vi "LCD.vi"(1 "stop":bool, 9 "Row 2":string, 10 "Row 1":string) -> ()   [LabVIEW 2017]
panel:
  out "error out":errorcluster
  in  "Back Light":bool
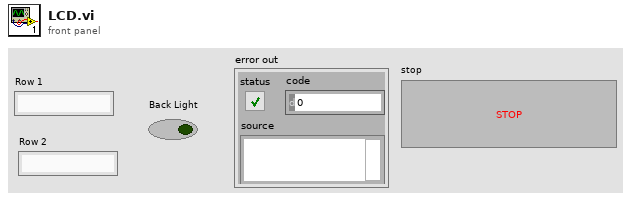
[diagram p1: front panel]
types:
  T1 = typedef "I2C.lvlib/I2C Reference.ctl" = cluster{"myRIO Reference":T2, "I2C Channels Enum":T6, "I2C Configuration":T7}
  T2 = typedef "myRIO Generic Hardware Reference.ctl" = cluster{"myRIO Model":T3, "myRIO Hardware Reference":T4}
  T3 = typedef "Hardware Version Enum.ctl" = enum16{"Unknown", "myRIO-1900", "myRIO-1950", "roboRIO", "NI ELVIS RIO CM"}
  T4 = typedef "myRIO v1.0 Reference.ctl" = cluster{"Generic FPGA Reference":T5, "Allow multiple opens":bool}
  T5 = typedef "Generic FPGA Reference.ctl" = refnum<k20>
  T6 = typedef "I2C Channels Enum.ctl" = enum16{"Not Connected", "A/I2C", "B/I2C", "I2C/I2C"}
  T7 = typedef "I2C.lvlib/I2C Configuration.ctl" = cluster{"I2C Transfer Rate":T8}
  T8 = typedef "I2C.lvlib/I2C Transfer Rate.ctl" = enum16{"Standard mode (100 kbps)", "Fast mode (400 kbps)"}
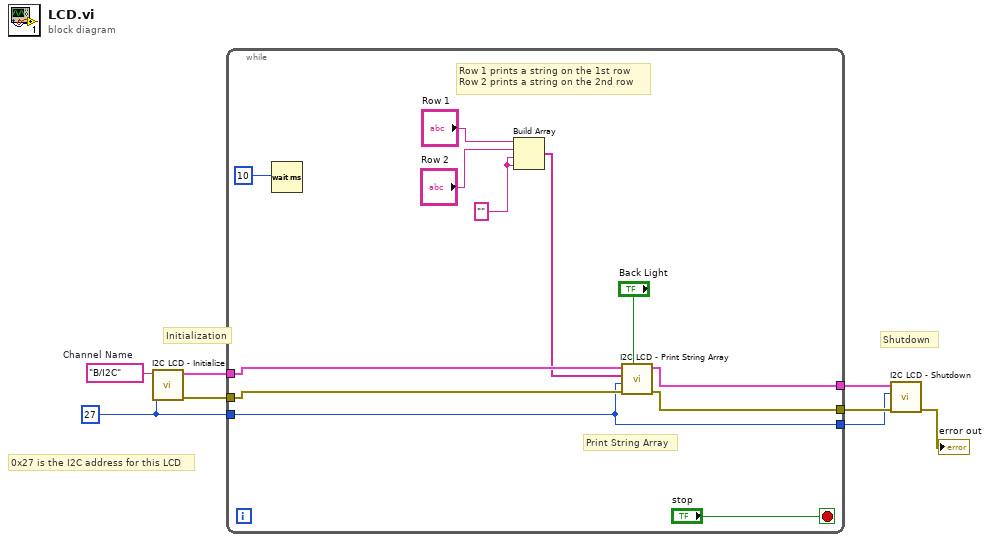
[diagram p0: block diagram]
diagram:
  w1 = tag "B/I2C"  # Channel Name
  w8 = u8 27 ("Slave Address (7-bit)")
  # "Initialization"
  # "Shutdown"
  # "0x27 is the I2C address for this LCD"
  n1 = call "I2C LCD - Initialize.vi"("Slave Address (7-bit)"=w8, "Channel Name"=w1) -> ("error out"=w7:errorcluster, "I2C Ref Out"=w6:T1)  [unwired: 8 in]
  n2 = while {
    tunnel: w8 -> [w16]
    tunnel: w7 -> [w20]
    tunnel: w6 -> [w18]
    tunnel: [w19] -> w5
    tunnel: [w17] -> w4
    tunnel: [w16] -> w3
    stop <- "stop" stop-if-true
    w11 = ""
    # "Row 1 prints a string on the 1st row\nRow 2 prints a string on the 2nd row"
    # "Print String Array"
    n3 = Wait (ms)(milliseconds to wait=10) -> ()  [unwired: 1 out]
    n4 = Build Array("Row 1", "Row 2", w11, w11) -> (w10:string[])
    n5 = call "I2C LCD - Print String Array.vi"("Back Light"="Back Light", "error in (no error)"=w20, "Slave Address (7-bit)"=w16, "String Array"=w10, "I2C Ref  in"=w18) -> ("error out"=w19:errorcluster, "I2C Ref Out"=w17:T1)  [unwired: 5 in]
  }
  n6 = call "I2C LCD - Shutdown.vi"("error in (no error)"=w5, "Slave Address (7-bit)"=w3, "I2C Ref Out"=w4) -> ("error out"=→"error out":errorcluster)  [unwired: 8 in]
